vi "Distort Image.vi"   [LabVIEW 2020, in "image.lvlib" / "ImageDistorter.lvclass"]
uses:
  ImageDistorter.lvclass
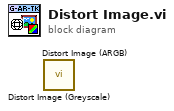
[diagram p0: block diagram]
diagram:
  n1 = call "Distort Image (Greyscale).vi"() -> ()  [unwired: 9 in, 3 out]
  n2 = call "Distort Image (ARGB).vi"() -> ()  [unwired: 9 in, 3 out]
